vi "To Default Value.vi"(10 "Ctl Refnum":refnum<vi>) -> ()   [LabVIEW 2024]
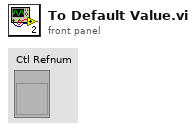
[diagram p1: front panel]
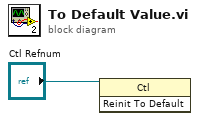
[diagram p0: block diagram]
diagram:
  n1 = invoke class="Ctl" method="Reinit To Default"(reference="Ctl Refnum") -> ()  [unwired: 2 in, 3 out]
